vi "Get_nearest_leaf_node.vi"(7 "Enum":enum16{"Search UP", "Search Down"}(ring), 10 "Row Number":i32, 11 "Tree Refnum":refnum<vi>) -> (2 "NOT Found Error":bool, 3 "Leaf Row Number OUT (Check if no error)":i32)   [LabVIEW 2012]
doc: "SciScan 1.2 160622"
panel:
  out "error out":errorcluster
  in  "error in (no error)":errorcluster
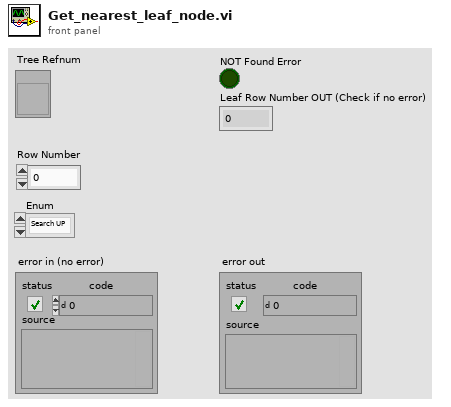
[diagram p1: front panel]
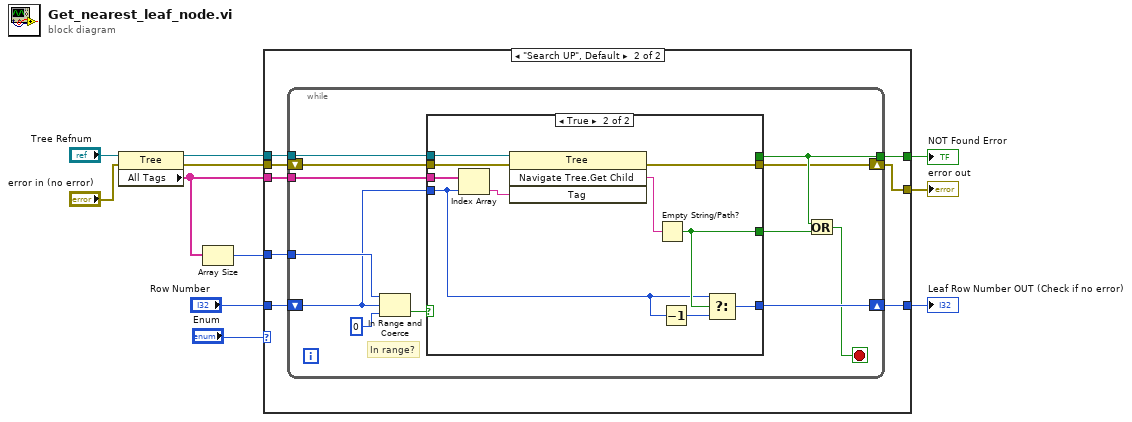
[diagram p0: block diagram]
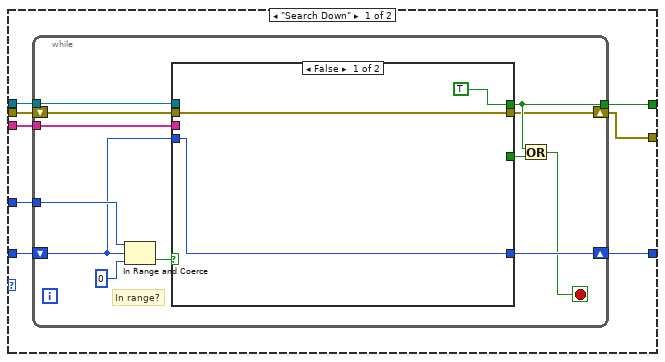
[diagram p2: hidden frame]
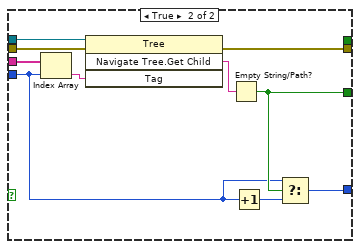
[diagram p3: hidden frame]
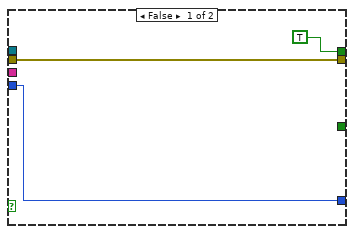
[diagram p4: hidden frame]
diagram:
  n1 = property class="Tree"(reference="Tree Refnum", error in="error in (no error)") -> (reference out=w8:refnum<vi>, error out=w2:errorcluster, "All Tags"=w7:string[])
  n2 = Array Size(array=w7) -> (size(s)=w6:i32)
  n3 = case shown="\"Search UP\", Default" "Enum" {
    tunnel: "Row Number" -> [w19 w52]
    tunnel: w8 -> [w18 w51]
    tunnel: w7 -> [w17 w50]
    tunnel: w6 -> [w16 w49]
    tunnel: [w15 w48] -> w5
    tunnel: [w14 w47] -> w4
    tunnel: w2 -> [w13 w46]
    tunnel: [w12 w45] -> w1
    frame "Search Down" {
      n4 = while {
        tunnel: w18 -> [w31]
        tunnel: w17 -> [w27]
        tunnel: w16 -> [w30]
        tunnel: [w26] -> w15
        shift-right: [w24] -> w14
        shift-left: w19 -> [w22]
        shift-right: [w20] -> w12
        shift-left: w13 -> [w21]
        stop <- w23 stop-if-true
        # "In range?"
        n5 = In Range and Coerce(upper limit=w30, x=w22, lower limit=0) -> (In Range?=w28:bool)  [unwired: 1 out]
        n6 = case shown="False" w28 {
          tunnel: w31 -> [_ w44]
          tunnel: [TRUE _] -> w26
          tunnel: w27 -> [_ w43]
          tunnel: w22 -> [w33 w38]
          tunnel: [_ w40] -> w25
          tunnel: [w33 w37] -> w24
          tunnel: w21 -> [w32 w36]
          tunnel: [w32 w35] -> w20
          frame False {
          }
          frame True {
            n7 = Index Array(array=w43, index=w38) -> (element=w42:string)
            n8 = invoke class="Tree" method="Navigate Tree.Get Child"(reference=w44, error in=w36, "Tag"=w42) -> (error out=w35:errorcluster, "Navigate Tree:Get Child"=w41:string)  [unwired: 1 in, 2 out]
            n9 = Empty String/Path?(string/path=w41) -> (empty?=w40:bool)
            n10 = Increment(x=w38) -> (x+1=w39:i32)
            n11 = Select(t=w38, s=w40, f=w39) -> (s? t:f=w37:i32)
          }
        }
        n12 = Or(x=w26, y=w25) -> (x .or. y?=w23:bool)
      }
    }
    frame "Search UP", Default {
      n13 = while {
        tunnel: w51 -> [w64]
        tunnel: w50 -> [w60]
        tunnel: w49 -> [w63]
        tunnel: [w59] -> w48
        shift-right: [w57] -> w47
        shift-left: w52 -> [w55]
        shift-right: [w53] -> w45
        shift-left: w46 -> [w54]
        stop <- w56 stop-if-true
        # "In range?"
        n14 = In Range and Coerce(upper limit=w63, x=w55, lower limit=0) -> (In Range?=w61:bool)  [unwired: 1 out]
        n15 = case shown="True" w61 {
          tunnel: w64 -> [_ w77]
          tunnel: [TRUE _] -> w59
          tunnel: w60 -> [_ w76]
          tunnel: w55 -> [w66 w71]
          tunnel: [_ w72] -> w58
          tunnel: [w66 w70] -> w57
          tunnel: w54 -> [w65 w69]
          tunnel: [w65 w68] -> w53
          frame False {
          }
          frame True {
            n16 = Index Array(array=w76, index=w71) -> (element=w75:string)
            n17 = invoke class="Tree" method="Navigate Tree.Get Child"(reference=w77, error in=w69, "Tag"=w75) -> (error out=w68:errorcluster, "Navigate Tree:Get Child"=w74:string)  [unwired: 1 in, 2 out]
            n18 = Empty String/Path?(string/path=w74) -> (empty?=w72:bool)
            n19 = Decrement(x=w71) -> (x-1=w73:i32)
            n20 = Select(t=w71, s=w72, f=w73) -> (s? t:f=w70:i32)
          }
        }
        n21 = Or(x=w59, y=w58) -> (x .or. y?=w56:bool)
      }
    }
  }
  "NOT Found Error" <- w5
  "Leaf Row Number OUT (Check if no error)" <- w4
  "error out" <- w1
